vi "ChannelList.vi"   [LabVIEW 2020, in "OXYGEN_Datastream.lvlib"]
uses:
  OXYGEN_Datastream.lvlib
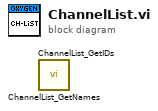
[diagram p0: block diagram]
diagram:
  n1 = call "ChannelList_GetNames.vi"() -> ()  [unwired: 8 in, 4 out]
  n2 = call "ChannelList_GetIDs.vi"() -> ()  [unwired: 8 in, 4 out]
